vi "solar_voy_def Import (Variants).vi"(6 "Suppress Errors? (T)":bool=TRUE, 8 "error in (no error)":errorcluster, 9 "TLMs":variant[](array[variant]), 10 "CMDs":variant[](array[variant]), 11 "TARGET":string) -> (0 "error out":errorcluster, 3 "PACKETS":T1[](array[typedef]) {"last_time" format="%<%H:%M:%S%3u %m/%d/%y>T"})   [LabVIEW 2018]
doc: "This imports Voyager command and telemetry packet definitions from LabVIEW variants. The variant should be a cluster packet and elements for each parameter/item. Use the followin arguments to modify each parameter/item via the label as '<label>,<arg0>,<arg1>'.\n\nLabel Modifiers:\nt=TYPE (block|string|int|uint|float) - Sets the COSMOS data type\nlv=LVTYPE (u8..u64,i8..i64,sgl,dbl,string,path,boolean,u16_enum,etc.) - Sets the LabVIEW data type\nb=BIT_SIZE - Sets the total parameter/item bit size\ne=EACH_BIT_SIZE - Sets the element bit size for string or block arrays only\ns=STATE|STATE - Sets the states starting at value 0:STATE|1:STATE|etc.\nd=DESC - Description of the item. MUST BE AT THE END OF THE LABEL.\nid - Sets the ID flag\n\nEx: MYITEM,b=1,lv=boolean,s=OK,ERROR, d=description"
uses:
  solar_voy_def_ctl ITEM TYPE.ctl
  type/solar_type Item Type.ctl
  solar_voy_def_ctl ITEM.ctl
  solar_voy_def_ctl PACKET.ctl
  solar_voy_def_ctl PACKET_ID.ctl
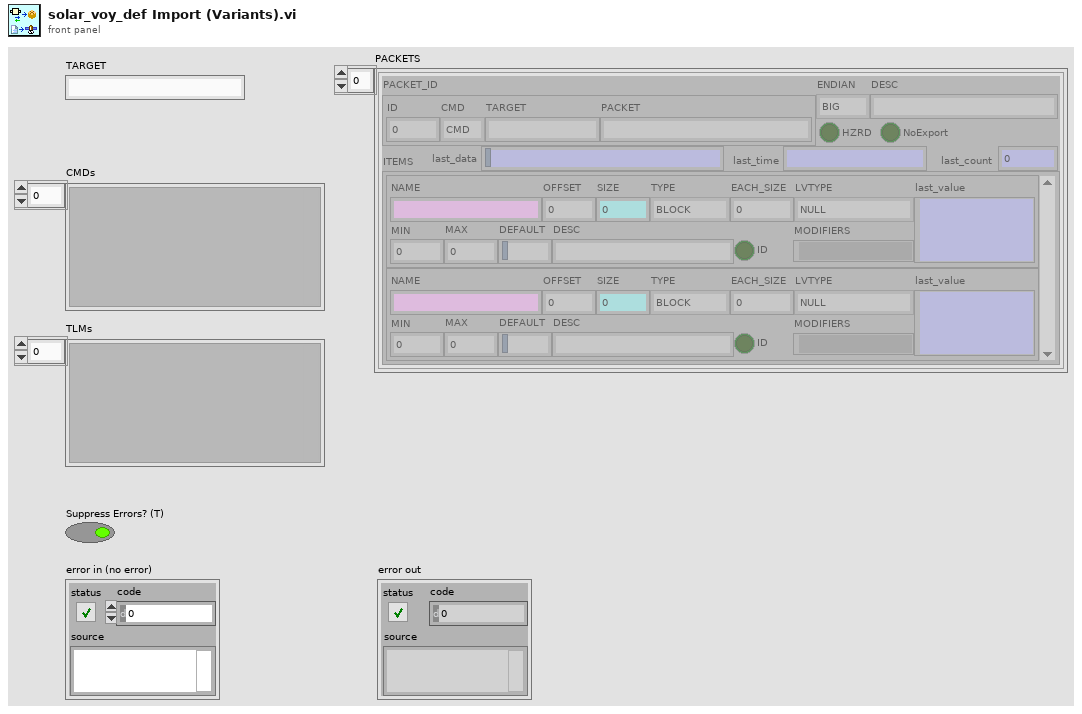
[diagram p1: front panel]
types:
  T1 = typedef "solar_voy_def_ctl PACKET.ctl" = cluster{"PACKET_ID":T2, "ENDIAN":enum8{"BIG", "LITTLE"}, "DESC":string, "HZRD":bool, "ITEMS":T3[], "NoExport":bool, "last_time":timestamp, "last_count":u32, "last_data":string}
  T2 = typedef "solar_voy_def_ctl PACKET_ID.ctl" = cluster{"ID":u16, "CMD":enum8{"CMD", "TLM"}, "TARGET":string, "PACKET":string}
  T3 = typedef "solar_voy_def_ctl ITEM.ctl" = cluster{"NAME":string, "OFFSET":i32, "SIZE":i32, "TYPE":T4, "EACH_SIZE":i32, "LVTYPE":T5, "MIN":dbl, "MAX":dbl, "DEFAULT":string, "DESC":string, "ID":bool, "MODIFIERS":variant, "last_value":variant}
  T4 = typedef "solar_voy_def_ctl ITEM TYPE.ctl" = enum8{"BLOCK", "INT", "UINT", "FLOAT", "STRING"}
  T5 = typedef "solar_type Item Type.ctl" = enum16{"NULL", "UNKNOWN", "CLUSTER", "I8", "I16", "I32", "I64", "U8", "U16", "U32", "U64", "U8_ENUM", "U16_ENUM", "U32_ENUM", "SGL", "DBL", "BOOLEAN", "STRING", "PATH", "VISA", "TAG", "TIME", "I8_1D", "I16_1D", "I32_1D", "I64_1D", "U8_1D", "U16_1D", "U32_1D", "U64_1D", "U8_ENUM_1D", "U16_ENUM_1D", "U32_ENUM_1D", "SGL_1D", "DBL_1D", "BOOLEAN_1D", "STRING_1D", "PATH_1D", "VISA_1D", "TAG_1D", "TIME_1D", "I8_2D", "I16_2D", "I32_2D", "I64_2D", "U8_2D", "U16_2D", "U32_2D", "U64_2D", "U8_ENUM_2D", "U16_ENUM_2D", "U32_ENUM_2D", "SGL_2D", "DBL_2D", "BOOLEAN_2D", "STRING_2D", "PATH_2D", "VISA_2D", "TAG_2D", "TIME_2D"}
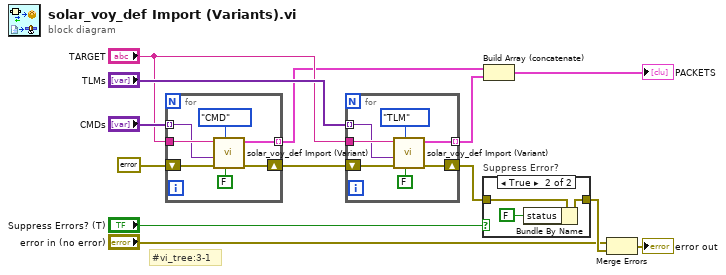
[diagram p0: block diagram]
diagram:
  # "#vi_tree:3-1"
  n1 = for {
    tunnel: "TARGET" -> [w17]
    shift-right: [w20] -> w7
    shift-left: errorcluster {"status"=FALSE, "code"=0, "source"=""} ("error in (no error)") -> [w19]
    tunnel: "CMDs" -> [w15] mode=indexing
    tunnel: [w14] -> w4 mode=indexing
    n2 = call "solar_voy_def Import (Variant).vi"("Suppress Errors? (T)"=FALSE, "CMD"=enum8{"CMD", "TLM"}."CMD", "error in (no error)"=w19, "Variant"=w15, "TARGET"=w17) -> ("error out"=w20:errorcluster, "PACKET"=w14:T1)  [unwired: 5 in]
  }
  n3 = for {
    tunnel: "TARGET" -> [w24]
    shift-right: [w27] -> w2
    shift-left: w7 -> [w26]
    tunnel: "TLMs" -> [w22] mode=indexing
    tunnel: [w21] -> w3 mode=indexing
    n4 = call "solar_voy_def Import (Variant).vi"("Suppress Errors? (T)"=FALSE, "CMD"=enum8{"CMD", "TLM"}."TLM", "error in (no error)"=w26, "Variant"=w22, "TARGET"=w24) -> ("error out"=w27:errorcluster, "PACKET"=w21:T1)  [unwired: 5 in]
  }
  n5 = case "Suppress Error?" shown="True" "Suppress Errors? (T)" {
    tunnel: w2 -> [w28 w31]
    tunnel: [w28 w30] -> w13
    frame False {
    }
    frame True {
      n6 = Bundle By Name(cluster=w31, "status"=FALSE) -> (w30:errorcluster)
    }
  }
  n7 = Build Array (concatenate)(w4, w3) -> (→"PACKETS":T1[])
  n8 = Merge Errors("error in (no error)", w13) -> (→"error out":errorcluster)
